vi "Check Client Status.vi"(8 "error in":errorcluster, 10 "client name":string, 11 "project ref in":refnum<vi>) -> (0 "error out":errorcluster, 1 "status":string, 2 "error message":string, 3 "project ref out":refnum<vi>)   [LabVIEW 2021, in "MeasurementClient Editor.lvlib"]
uses:
  MeasurementClient Editor.lvlib
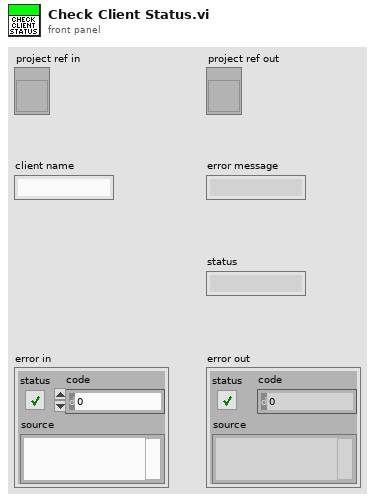
[diagram p1: front panel]
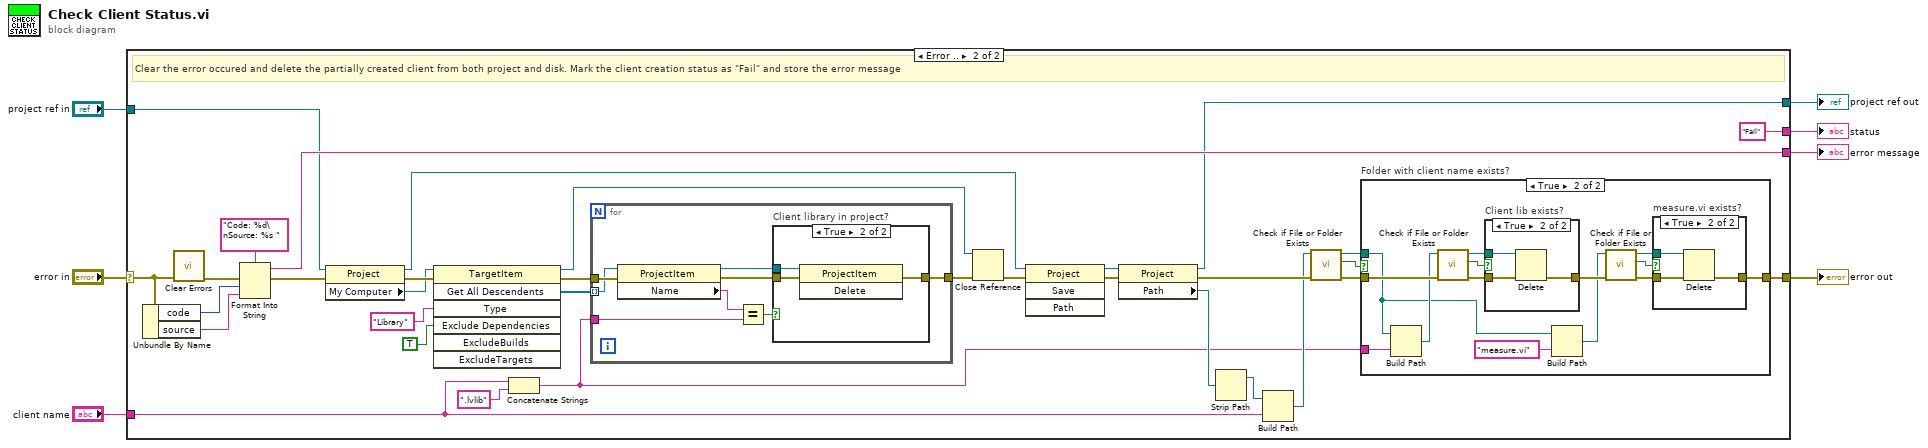
[diagram p0: block diagram]
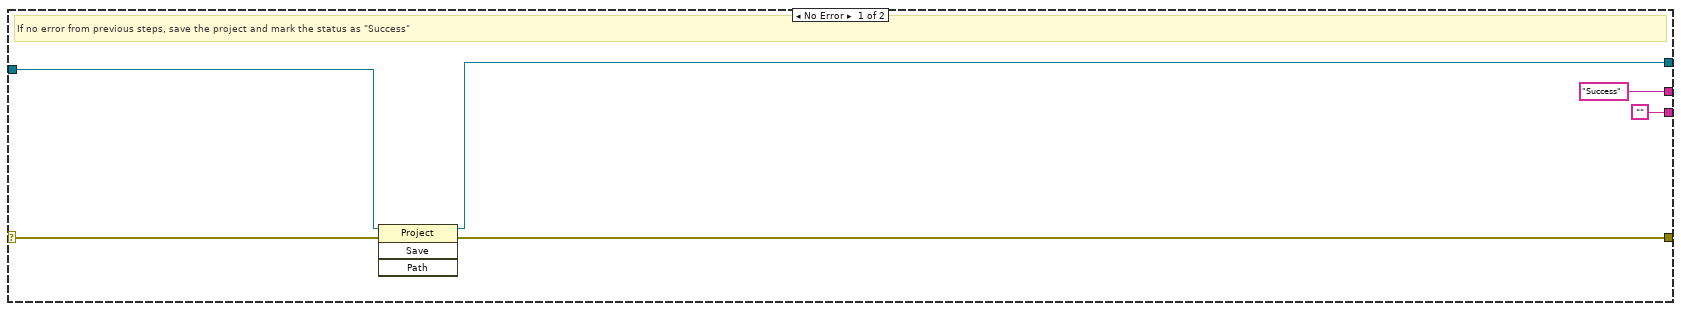
[diagram p2: hidden frame]
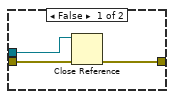
[diagram p3: hidden frame]
diagram:
  n1 = case shown="Error .." "error in" {
    selector: "error in" -> [w13 w32]
    tunnel: [w10 w23] -> w7
    tunnel: "project ref in" -> [w12 w41]
    tunnel: [w11 w28] -> w4
    tunnel: ["Success" "Fail"] -> w3
    tunnel: ["" w42] -> w2
    tunnel: "client name" -> [_ w16]
    frame No Error {
      # "If no error from previous steps, save the project and mark the status as \"Success\""
      n2 = invoke class="Project" method="Save"(reference=w12, error in=w13) -> (reference out=w11:refnum<vi>, error out=w10:errorcluster)  [unwired: 2 in, 2 out]
    }
    frame Error {
      # "Clear the error occured and delete the partially created client from both project and disk. Mark the client creation status as \"Fail\" and store the error message"
      n3 = Unbundle By Name(w32) -> ("code"=w44:i32, "source"=w43:string)
      n4 = call <vilib>:"Clear Errors.vi"("error in (no error)"=w32) -> ("error out"=w33:errorcluster)  [unwired: 5 in, 1 out]
      n5 = Format Into String(format string="Code: %d\nSource: %s ", error in=w33, w44, w43) -> (resulting string=w42:string, error out=w45:errorcluster)  [unwired: 1 in]
      n6 = property class="Project"(reference=w41, error in=w45) -> (reference out=w19:refnum<vi>, error out=w40:errorcluster, "My Computer"=w39:refnum<vi>)
      n7 = invoke class="TargetItem" method="Get All Descendents"(reference=w39, error in=w40, "Type"="Library", "Exclude Dependencies"=TRUE ("ExcludeDependencies")) -> (reference out=w30:refnum<vi>, error out=w36:errorcluster, "All Descendents"=w35:refnum<vi>[])  [unwired: 3 in, 4 out]
      n8 = Concatenate Strings(w16, ".lvlib" ("string")) -> (w15:string)
      n9 = for {
        tunnel: w36 -> [w54]
        tunnel: w35 -> [w53] mode=indexing
        tunnel: w15 -> [w51]
        tunnel: [w47] -> w34
        n10 = property class="ProjectItem"(reference=w53, error in=w54) -> (reference out=w50:refnum<vi>, error out=w48:errorcluster, "Name"=w52:string)
        n11 = Equal?(x=w52, y=w51) -> (x = y?=w49:bool)
        n12 = case "Client library in project?" shown="True" w49 {
          tunnel: w50 -> [w55 w60]
          tunnel: w48 -> [w57 w59]
          tunnel: [w56 w58] -> w47
          frame False {
            n13 = Close Reference(reference=w55, error in (no error)=w57) -> (error out=w56:errorcluster)
          }
          frame True {
            n14 = invoke class="ProjectItem" method="Delete"(reference=w60, error in=w59) -> (error out=w58:errorcluster)  [unwired: 1 in, 2 out]
          }
        }
      }
      n15 = Close Reference(reference=w30, error in (no error)=w34) -> (error out=w31:errorcluster)
      n16 = invoke class="Project" method="Save"(reference=w19, error in=w31) -> (reference out=w18:refnum<vi>, error out=w20:errorcluster)  [unwired: 2 in, 2 out]
      n17 = property class="Project"(reference=w18, error in=w20) -> (reference out=w28:refnum<vi>, error out=w29:errorcluster, "Path"=w27:path)
      n18 = Strip Path(path=w27) -> (stripped path=w26:path)  [unwired: 1 out]
      n19 = Build Path(base path=w26, name or relative path=w16) -> (appended path=w25:path)
      n20 = call <vilib>:"Check if File or Folder Exists.vi"("error in (no error)"=w29, "path"=w25) -> ("error out"=w24:errorcluster, "file or folder exists?"=w14:bool, "dup path"=w22:path)  [unwired: 7 in]
      n21 = case "Folder with client name exists?" shown="True" w14 {
        tunnel: w24 -> [w61 w75]
        tunnel: [w61 w63] -> w23
        tunnel: w22 -> [_ w69]
        tunnel: w15 -> [_ w74]
        frame False {
        }
        frame True {
          n22 = Build Path(base path=w69, name or relative path=w74) -> (appended path=w73:path)
          n23 = call <vilib>:"Check if File or Folder Exists.vi"("error in (no error)"=w75, "path"=w73) -> ("error out"=w72:errorcluster, "file or folder exists?"=w71:bool, "dup path"=w70:path)  [unwired: 7 in]
          n24 = case "Client lib exists?" shown="True" w71 {
            tunnel: w72 -> [w80 w83]
            tunnel: w70 -> [_ w81]
            tunnel: [w80 w82] -> w64
            frame False {
            }
            frame True {
              n25 = Delete(path (use dialog)=w81, error in=w83) -> (error out=w82:errorcluster)  [unwired: 3 in, 2 out]
            }
          }
          n26 = Build Path(base path=w69, name or relative path="measure.vi") -> (appended path=w62:path)
          n27 = call <vilib>:"Check if File or Folder Exists.vi"("error in (no error)"=w64, "path"=w62) -> ("error out"=w65:errorcluster, "file or folder exists?"=w66:bool, "dup path"=w67:path)  [unwired: 7 in]
          n28 = case "measure.vi exists?" shown="True" w66 {
            tunnel: w65 -> [w76 w79]
            tunnel: w67 -> [_ w77]
            tunnel: [w76 w78] -> w63
            frame False {
            }
            frame True {
              n29 = Delete(path (use dialog)=w77, error in=w79) -> (error out=w78:errorcluster)  [unwired: 3 in, 2 out]
            }
          }
        }
      }
    }
  }
  "project ref out" <- w4
  "error out" <- w7
  "status" <- w3
  "error message" <- w2
